vi "Reset.vi"(0 "VisaCluster":T1, 11 "error in (no error)":errorcluster) -> (4 "VisaCluster":T1, 8 "Answer":string, 15 "error out":errorcluster)   [LabVIEW 2014, in "FH 55.lvlib"]
doc: "The VI starts the function Reset. Max/Min or Peak sets to Zero.\n\n Durch die Funktion Reset wird MAX/MIN bzw. Peak auf Null gesetzt."
uses:
  FH 55.lvlib
  TypeDef/VisaCluster.ctl
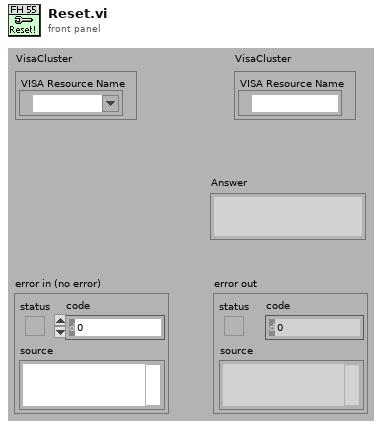
[diagram p1: front panel]
types:
  T1 = typedef "FH 55.lvlib/VisaCluster.ctl" = cluster{"VISA Resource Name":refnum<visa-resource-name>}
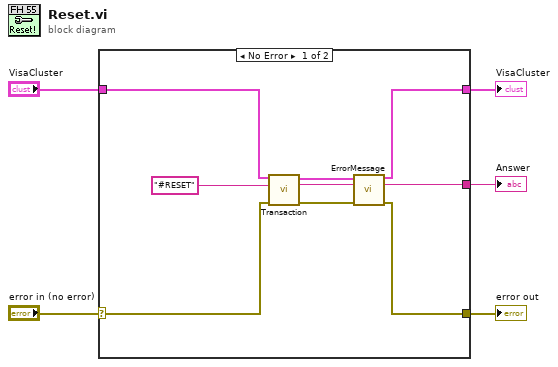
[diagram p0: block diagram]
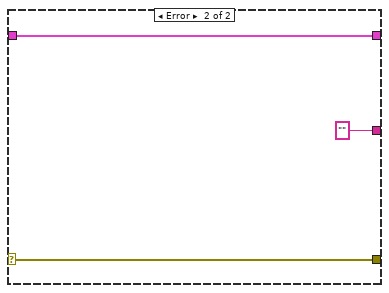
[diagram p2: hidden frame]
diagram:
  n1 = case shown="No Error" "error in (no error)" {
    selector: "error in (no error)" -> [w10 w16]
    tunnel: "VisaCluster" -> [w11 w17]
    tunnel: [w14 w17] -> w1
    tunnel: [w12 w16] -> w3
    tunnel: [w13 ""] -> w2
    frame No Error {
      n2 = call "Transaction.vi"("VisaCluster"=w11, "Command"="#RESET", "error in (no error)"=w10) -> ("VisaCluster"=w7:T1, "Answer"=w8:string, "error out"=w9:errorcluster)  [unwired: 9 in, 1 out]
      n3 = call "ErrorMessage.vi"("VisaCluster"=w7, "Message In"=w8, "error in (no error)"=w9) -> ("VisaCluster"=w14:T1, "Message Out"=w13:string, "error out"=w12:errorcluster)  [unwired: 10 in]
    }
    frame Error {
    }
  }
  "error out" <- w3
  "Answer" <- w2
  "VisaCluster" <- w1
